vi "Decode packed double.vi"(10 "Wire Type":T1=enum."I64", 11 "Data":u8[](array[numeric]) format="%.0x") -> (2 "error out":errorcluster, 3 "double":dbl[](array[numeric]))   [LabVIEW 2020, in "LV-Proto.lvlib"]
uses:
  LV-Proto.lvlib
  Wire Type.ctl
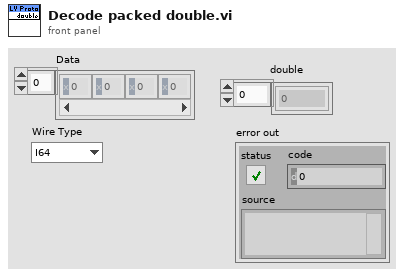
[diagram p1: front panel]
types:
  T1 = typedef "LV-Proto.lvlib/Wire Type.ctl" = enum8{"VARINT", "I64", "LEN", "SGROUP (Deprecated)", "EGROUP (Deprecated)", "I32"}
  T2 = enum16{"big-endian, network order", "native, host order", "little-endian"}
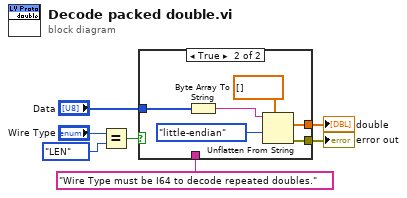
[diagram p0: block diagram]
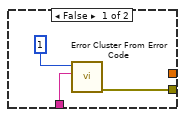
[diagram p2: hidden frame]
diagram:
  n1 = Equal?(x="Wire Type", y=Wire_Type."LEN") -> (x = y?=w3:bool)
  n2 = case shown="True" w3 {
    tunnel: "Data" -> [_ w16]
    tunnel: [_ w13] -> w6
    tunnel: [w10 w12] -> w2
    tunnel: "Wire Type must be I64 to decode repeated doubles." -> [w8 _]
    frame False {
      n3 = call <vilib>:"Error Cluster From Error Code.vi"("error message (\"\")"=w8, "error code (0)"=1) -> ("error out"=w10:errorcluster)  [unwired: 7 in]
    }
    frame True {
      n4 = Byte Array To String(unsigned byte array=w16) -> (string=w11:string)
      n5 = Unflatten From String(type=dbl[] [], binary string=w11, byte order (0:big-endian, network order)=T2."little-endian") -> (value=w13:dbl[], error out=w12:errorcluster)  [unwired: 2 in, 1 out]
    }
  }
  "double" <- w6
  "error out" <- w2
